vi "8HP_Convert serial string to Eng vals.vi"(0 "Serial buffer string (excluding FrameChar)":string) -> (11 "All vals":sgl[](array[numeric]), 12 "Pressures":sgl[][](graph), 13 "Gyration vector (deg / s)":sgl[](array[numeric]), 14 "External thermistor 0 temperature (°C)":sgl, 15 "External thermistor 1 temperature (°C)":sgl, 16 "Atmospheric pressure (mbar)":sgl, 17 "Env. sensor die temperature (°C)":sgl, 18 "Relative humidity (%)":sgl, 19 "Acceleration vector (g)":sgl[](array[numeric]))   [LabVIEW 2020]
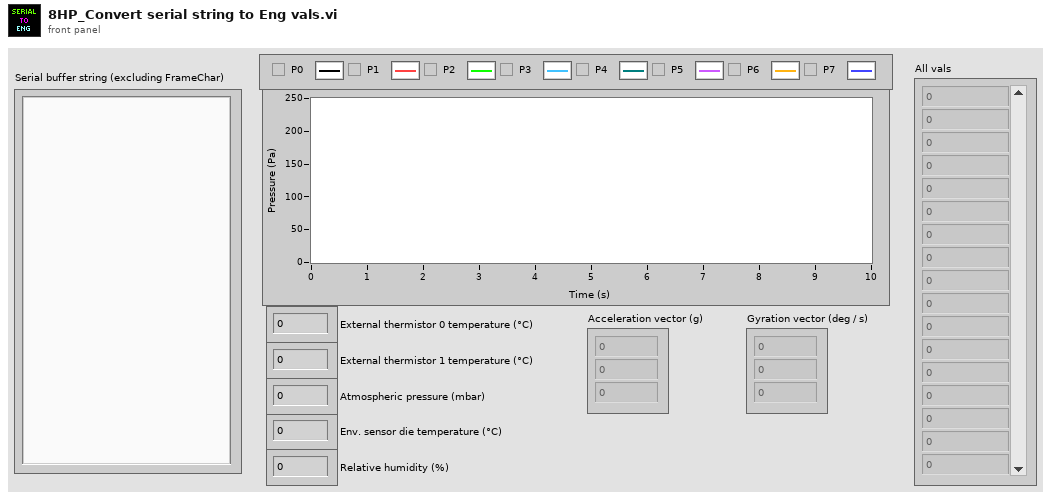
[diagram p1: front panel]
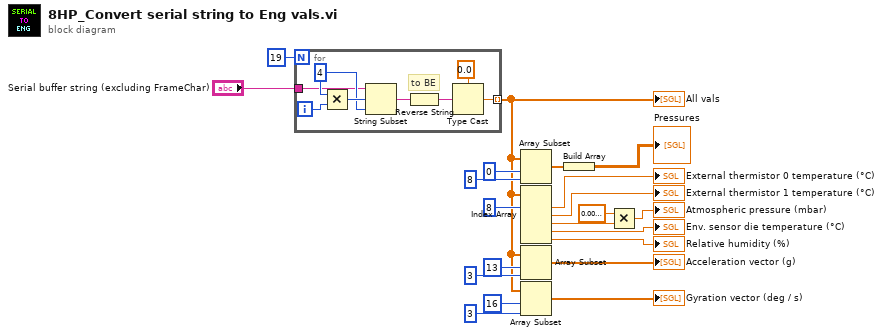
[diagram p0: block diagram]
diagram:
  n1 = for {
    N: 19 -> [_]
    tunnel: [w23] -> w1 mode=indexing
    tunnel: "Serial buffer string (excluding FrameChar)" -> [w22]
    i -> [w29]
    w27 = 4 ("x")
    # "to BE"
    n2 = Multiply(x=w27, y=w29) -> (x*y=w28:i32)
    n3 = String Subset(string=w22, offset (0)=w28, length (rest)=w27) -> (substring=w26:string)
    n4 = Reverse String(1:w26) -> (0:w25:string)
    n5 = Type Cast(type=sgl 0.0 ("byte count"), x=w25) -> (*(type *) &x=w23:sgl)
  }
  "All vals" <- w1
  n6 = Array Subset(array=w1, index=0, length=8) -> (w17:sgl[])
  n7 = Index Array(array=w1, index #1=8 ("index")) -> (element #1=→"External thermistor 0 temperature (°C)":sgl, element #2=→"External thermistor 1 temperature (°C)":sgl, element #3=w4:sgl, element #4=→"Env. sensor die temperature (°C)":sgl, element #5=→"Relative humidity (%)":sgl)  [unwired: 4 in]
  n8 = Array Subset(array=w1, index=13, length=3) -> (→"Acceleration vector (g)":sgl[])
  n9 = Array Subset(array=w1, index=16, length=3) -> (→"Gyration vector (deg / s)":sgl[])
  n10 = Build Array(w17) -> (→"Pressures":sgl[][])
  n11 = Multiply(x=sgl 0.01, y=w4) -> (x*y=→"Atmospheric pressure (mbar)":sgl)
